vi "Sprachumschaltung.vi"(8 "Fehler (Eingang, kein Fehler)":errorcluster, 10 "menu reference":refnum<k9>, 11 "Cluster (Eingang)":refnum<vi>) -> (0 "Fehler (Ausgang)":errorcluster)   [LabVIEW 2020, in "allgemeine Sub-VIs.lvlib"]
uses:
  allgemeine Sub-VIs.lvlib
  Stoerungen/FGV Stoerungsdatei Aktionen.ctl
  Funktionstasten/Zustaende.ctl
  PNS/Komm Modbus/Aktionen FGV Komm MB.ctl
  Seiten/System Einstellungen V2/Aktioen FGV System Konstanten.ctl
  SysLog/SysLog Interface.ctl
  Sprachverwaltung/Sprachverwaltung.lvlib
  Stoerungen/Stoerungen.lvlib
  Funktionstasten/Funktionstasten.lvlib
  PNS/Komm Modbus/Komm Modbus.lvlib
  PNS/Komm Modbus/Modbus TypDef.lvlib
  SysLog/SysLog.lvlib
  Seiten/System Einstellungen V2/System Einstellungen V2.lvlib
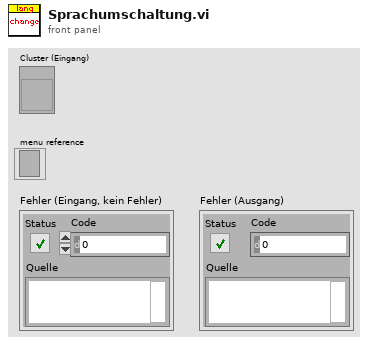
[diagram p1: front panel]
types:
  T1 = typedef "System Einstellungen V2.lvlib/Aktioen FGV System Konstanten.ctl" = enum16{"lesen", "laden", "speichern", "Sprache"}
  T2 = typedef "PNS.lvlib/Komm Modbus.lvlib/Modbus TypDef.lvlib/Aktionen FGV Komm MB.ctl" = enum16{"initialisieren", "lesen", "Verbindung herstellen", "Verbindung beenden", "Komm Modbus", "Sollwerte vorgeben", "change lang"}
  T3 = typedef "Funktionstasten.lvlib/Zustaende.ctl" = enum16{"Standby", "Pause", "Eco", "Messen", "Kalibrieren", "Spülen Filter", "Spülen Leitung", "Umgebungsluft", "0-Gas", "Cal-Gas", "CG zu PNS", "-------------", "Init 1", "Init 2", "Init 3", "Init 4", "Messen vorbereiten", "Messen durchführen", "Exit"}
  T4 = typedef "Stoerungen.lvlib/FGV Stoerungsdatei Aktionen.ctl" = enum16{"lesen", "laden", "Neue Werte"}
  T5 = typedef "SysLog.lvlib/SysLog Interface.ctl" = cluster{"FehlermeldungsCode":i32, "ErfolgsmeldungsCode":i32, "ParameterListenString":string, "Anzeige":bool, "SysLogIcon":enum16{"OK", "Warnung", "Fehler"}, "intern":bool}
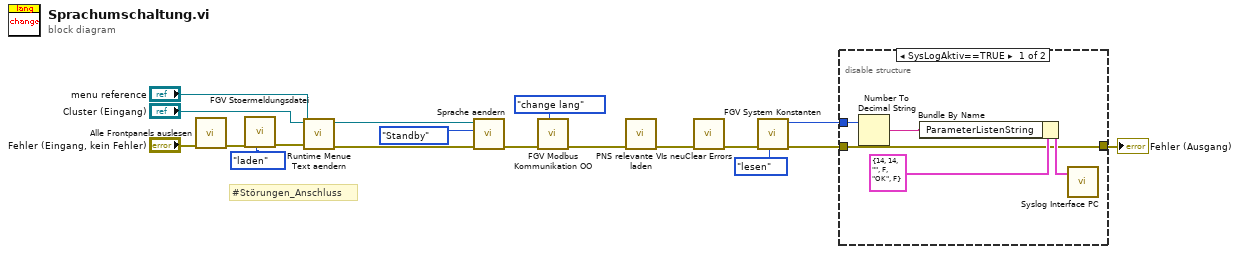
[diagram p0: block diagram]
diagram:
  # "#Störungen_Anschluss"
  n1 = call "Alle Frontpanels auslesen.vi"("Fehler (Eingang, kein Fehler)"="Fehler (Eingang, kein Fehler)") -> ("Fehler (Ausgang)"=w8:errorcluster)  [unwired: 10 in]
  n2 = call "FGV Stoermeldungsdatei.vi"("Aktionen"=FGV_Stoerungsdatei_Aktionen."laden", "Fehler (Eingang, kein Fehler)"=w8) -> ("Fehler (Ausgang)"=w7:errorcluster)  [unwired: 4 in, 5 out]
  n3 = call "Runtime Menue Text aendern.vi"("Fehler (Eingang, kein Fehler)"=w7, "Menüreferenz"="menu reference") -> ("Fehler (Ausgang)"=w6:errorcluster)  [unwired: 9 in]
  n4 = call "Sprache aendern.vi"("Fehler (Eingang, kein Fehler)"=w6, "Zustand"=Zustaende."Standby", "Cluster (Eingang)"="Cluster (Eingang)") -> ("error out"=w5:errorcluster)  [unwired: 7 in, 1 out]
  n5 = call "FGV Modbus Kommunikation OO.vi"("Aktionen"=Aktionen_FGV_Komm_MB."change lang", "error in"=w5) -> ("Fehler (Ausgang)"=w12:errorcluster)  [unwired: 3 in, 4 out]
  n6 = call "PNS relevante VIs neu laden.vi"("Fehler (Eingang, kein Fehler)"=w12) -> ("Fehler (Ausgang)"=w11:errorcluster)  [unwired: 10 in]
  n7 = call <vilib>:"Clear Errors.vi"("error in (no error)"=w11) -> ("error out"=w3:errorcluster)  [unwired: 5 in, 1 out]
  n8 = call "FGV System Konstanten.vi"("Aktionen"=Aktioen_FGV_System_Konstanten."lesen", "error in"=w3) -> ("error out"=w2:errorcluster, "Sprachindex"=w9:u16)  [unwired: 5 in, 3 out]
  n9 = disable-structure shown="SysLogAktiv==TRUE" {
    disable-tunnel: w9 -> [w22 _]
    disable-tunnel: w2 -> [w18 w23]
    disable-tunnel: [w18 _] -> w1
    disable-tunnel: [_ w23] -> _
    frame condition #0 (active) {
      n10 = Number To Decimal String(number=w22) -> (decimal integer string=w19:string)  [unwired: 1 in]
      n11 = Bundle By Name(cluster=T5 {"FehlermeldungsCode"=14, "ErfolgsmeldungsCode"=14, "ParameterListenString"="", "Anzeige"=FALSE, "SysLogIcon"=enum."OK", "intern"=FALSE} ("Cluster (in)"), "ParameterListenString"=w19) -> (w20:T5)
      n12 = call "Syslog Interface PC.vi"("Cluster (in)"=w20) -> ()  [unwired: 10 in, 1 out]
    }
    frame condition #1 {
    }
  }
  "Fehler (Ausgang)" <- w1
